vi "Plot XY SM.vi"(0 "Init Plot Cluster":T1={"Y Scale Label Left"="left", "Y Scale Label Right"="right", "X Scale Label"="Time", "Ymin Left"=0.0, "Ymax Left"=1.0, "Ymin Right"=-5.0, "Ymax Right"=5.0, "Number of Left Data"=0, "PlotNames Array"=["Temp1", "Temp2", "Temp3", "Temp4", "Temp5", "Temp6", "Temp7"]}, 2 "Mode":T2, 5 "Add Time":dbl, 7 "Add Data":dbl[](array[numeric])) -> (4 "Plot":cluster{dbl[], dbl[]}[](graph))   [LabVIEW 2014]
uses:
  Dryer Performance/Graph Mode Control.ctl
panel:
  in  "Array":bool[](array[boolean])
  in  "OK":bool
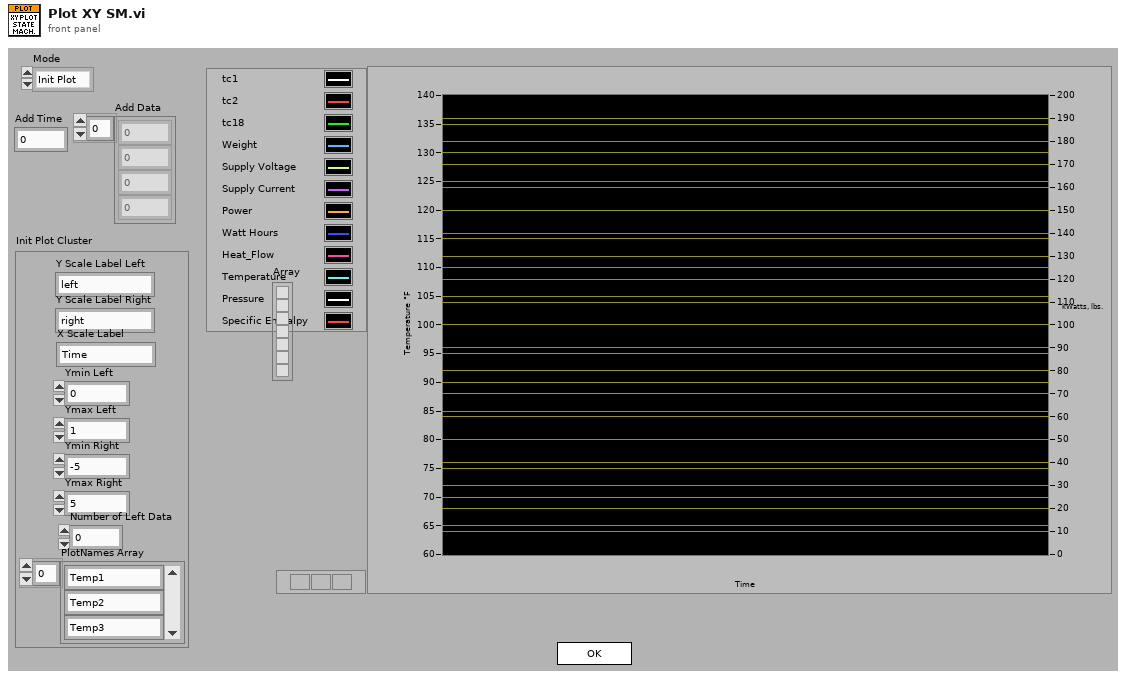
[diagram p1: front panel]
types:
  T1 = cluster{"Y Scale Label Left":string, "Y Scale Label Right":string, "X Scale Label":string, "Ymin Left":dbl, "Ymax Left":dbl, "Ymin Right":dbl, "Ymax Right":dbl, "Number of Left Data":u8, "PlotNames Array":string[]}
  T2 = typedef "Graph Mode Control.ctl" = enum16{"Init Plot", "Add Data", "Simulate"}
  T3 = enum32{"invalid app kind", "Development System", "Run Time System", "Student Edition", "Embedded LabVIEW", "Evaluation", "Custom"}
  T4 = enum32{"Invalid", "Standard", "Closed", "Hidden", "Minimized", "Maximized"}
  T5 = cluster{"Core":cluster{"Current VI Reference":refnum<vi>, "Close Panel on Exit?":bool}, "Num Plots":u32, "Time Array":dbl[], "Data Array":dbl[][], "New Time":dbl, "New Data":dbl[]}
  T6 = cluster{"Current VI Reference":refnum<vi>, "Close Panel on Exit?":bool}
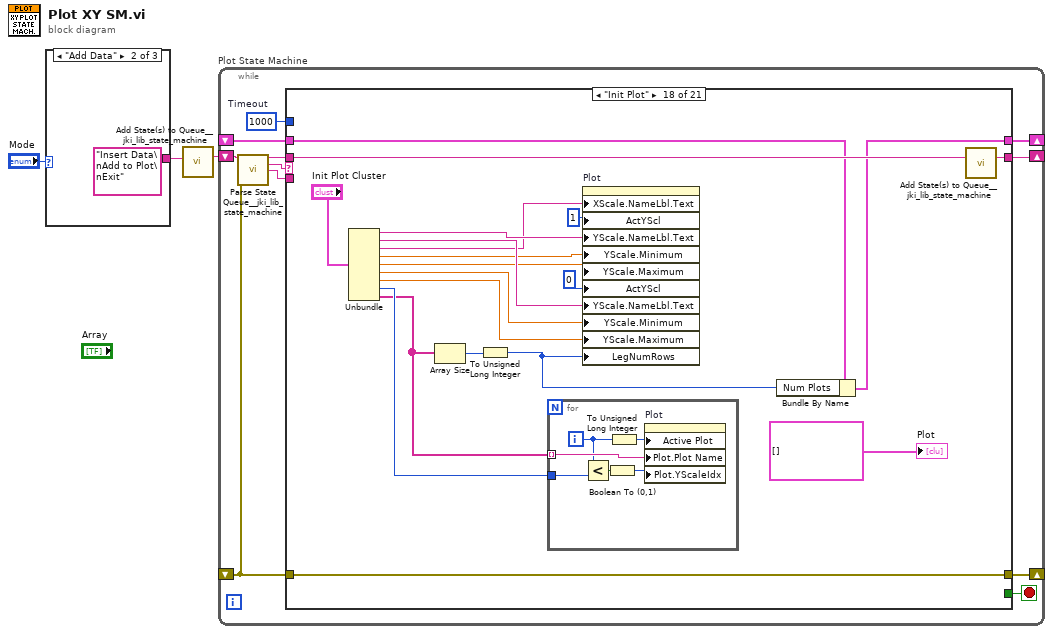
[diagram p0: block diagram]
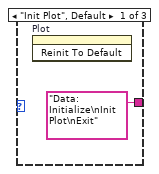
[diagram p2: hidden frame]
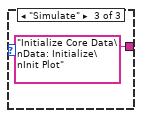
[diagram p3: hidden frame]
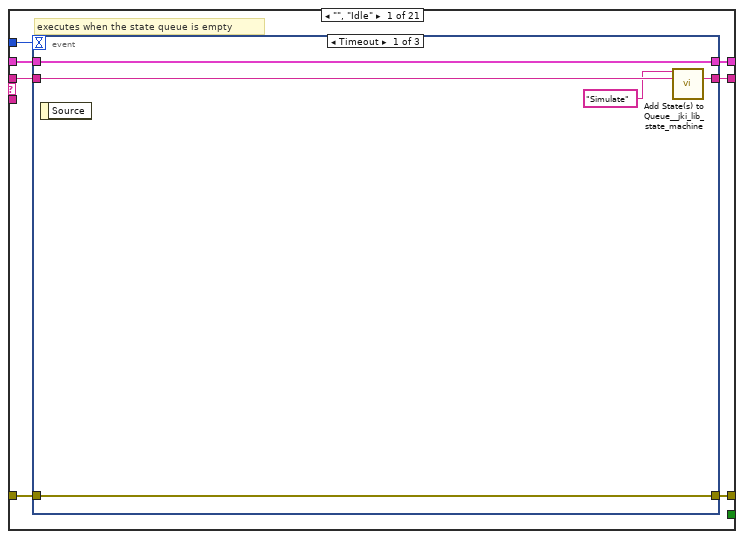
[diagram p4: hidden frame]
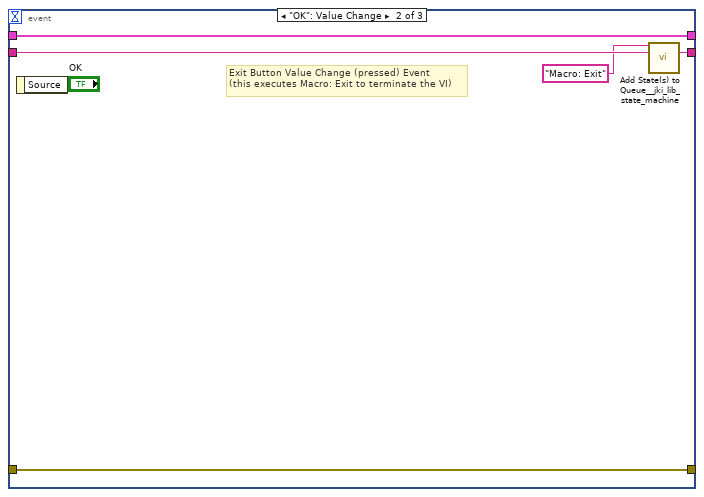
[diagram p5: hidden frame]
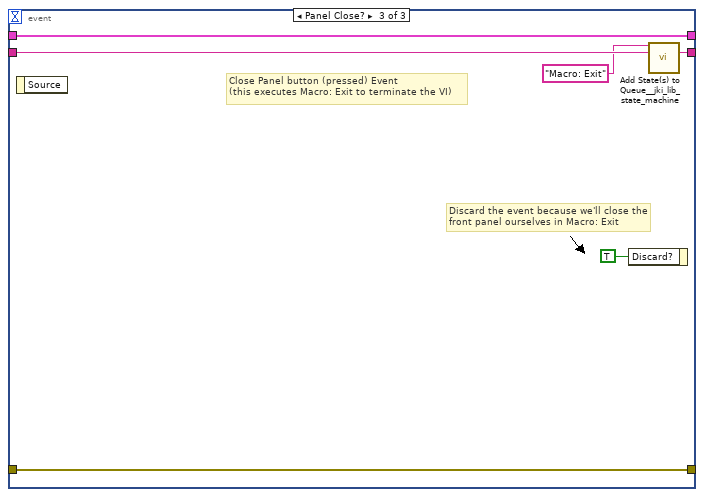
[diagram p6: hidden frame]
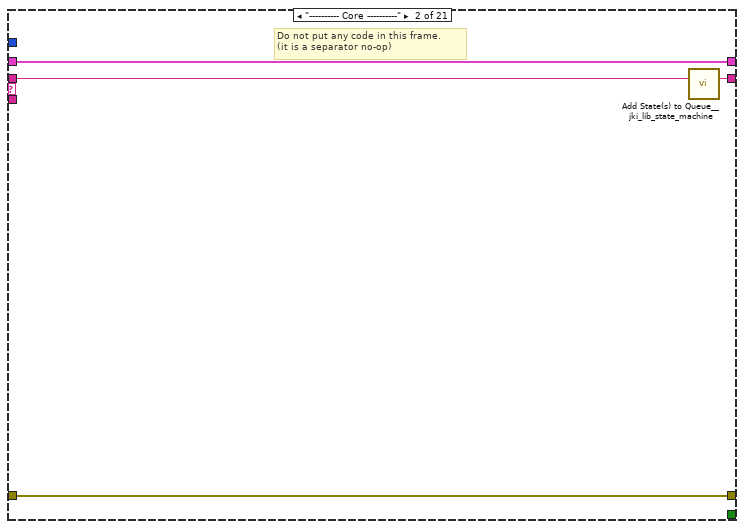
[diagram p7: hidden frame]
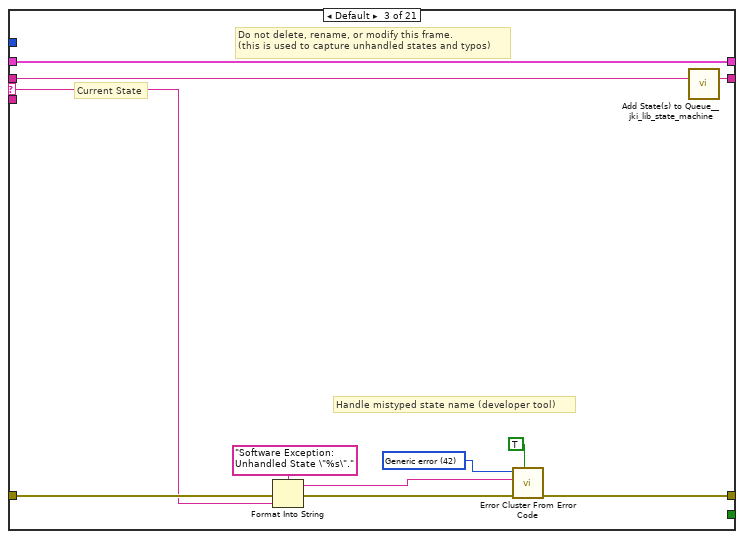
[diagram p8: hidden frame]
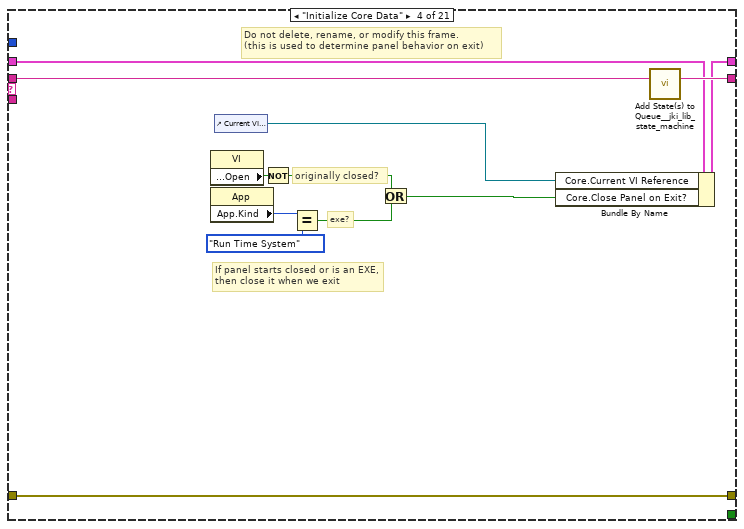
[diagram p9: hidden frame]
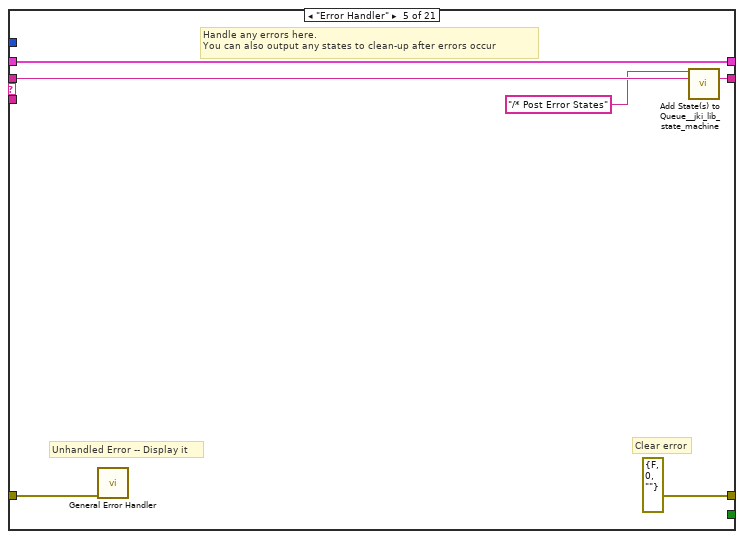
[diagram p10: hidden frame]
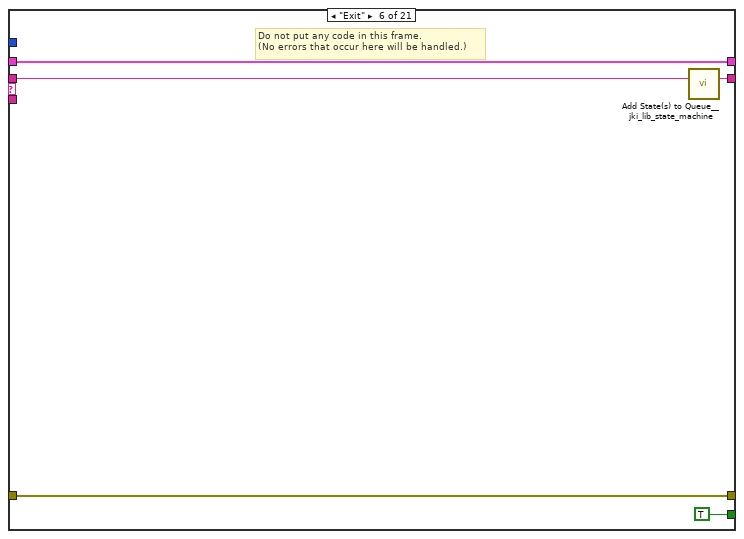
[diagram p11: hidden frame]
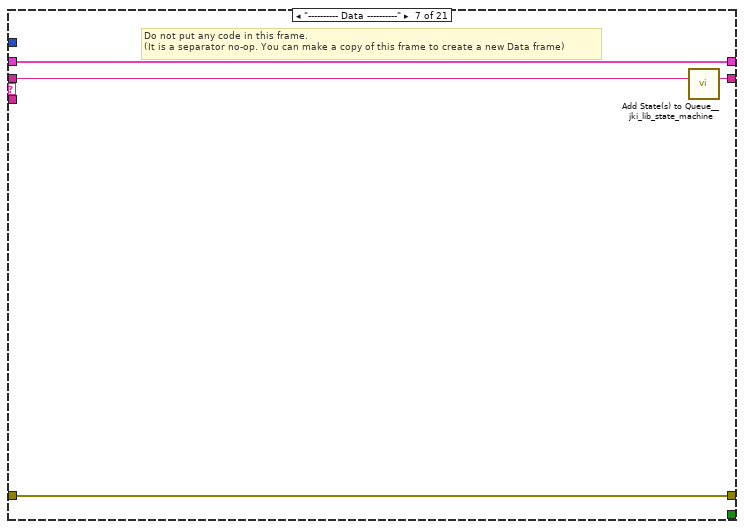
[diagram p12: hidden frame]
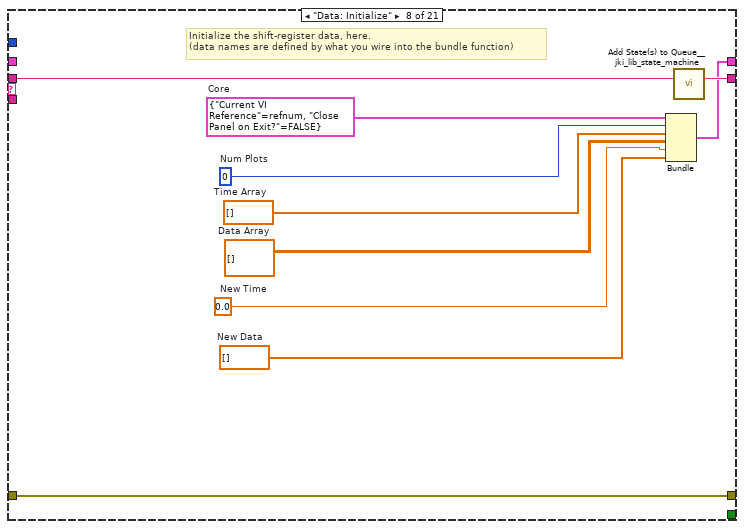
[diagram p13: hidden frame]
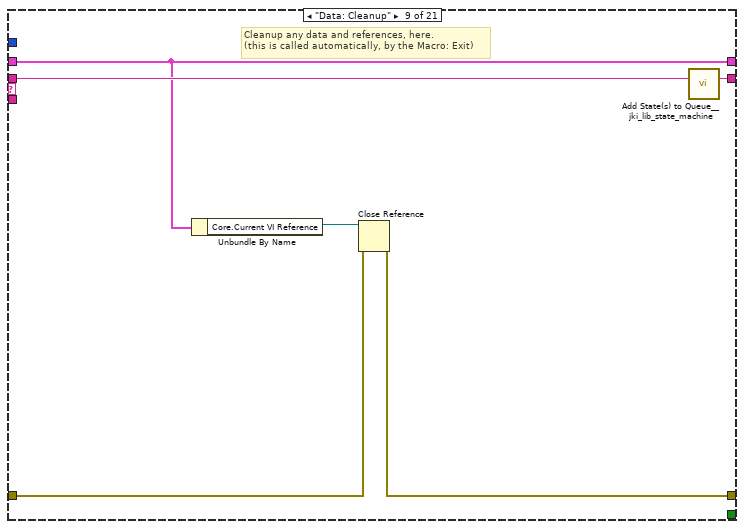
[diagram p14: hidden frame]
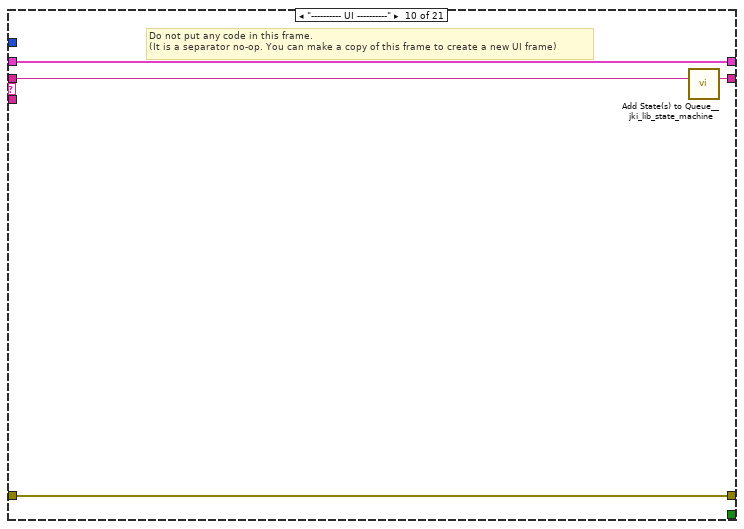
[diagram p15: hidden frame]
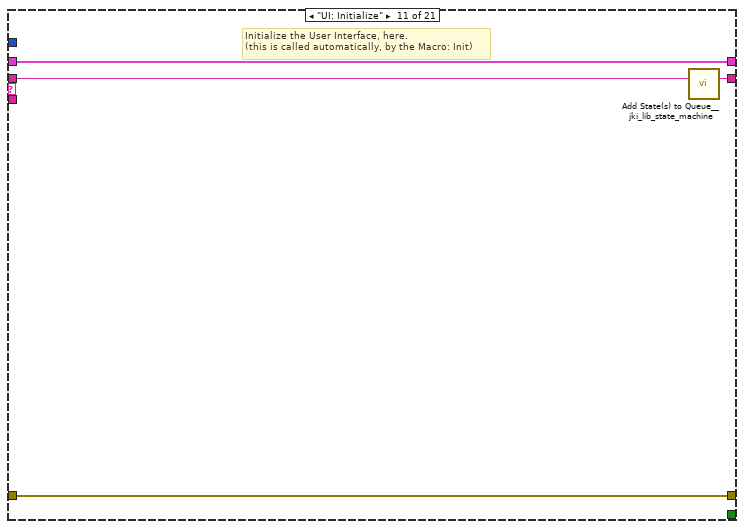
[diagram p16: hidden frame]
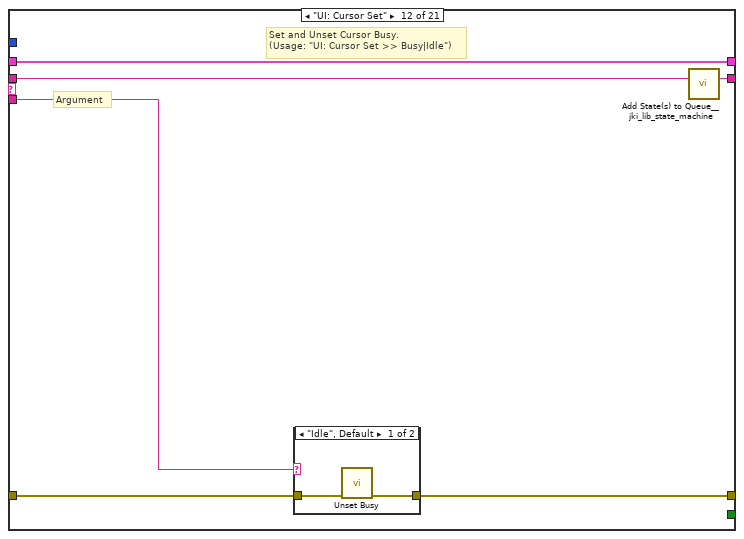
[diagram p17: hidden frame]
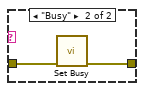
[diagram p18: hidden frame]
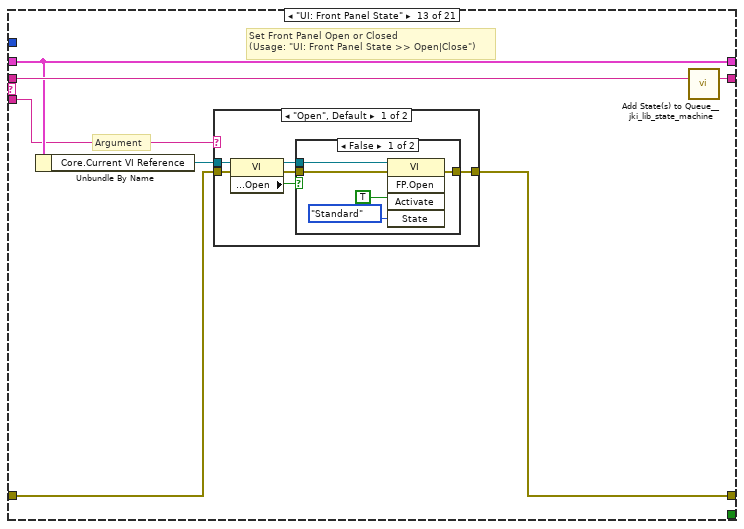
[diagram p19: hidden frame]
diagram:
  n1 = case shown="\"Add Data\"" "Mode" {
    tunnel: ["Data: Initialize\nInit Plot\nExit" "Insert Data\nAdd to Plot\nExit" "Initialize Core Data\nData: Initialize\nInit Plot"] -> w2
    frame "Init Plot", Default {
      n2 = invoke on="Plot" class="XYGraph (strict)" method="Reinit To Default"() -> ()  [unwired: 3 in, 3 out]
    }
    frame "Add Data" {
    }
    frame "Simulate" {
    }
  }
  n3 = call <vilib>:"Add State(s) to Queue__jki_lib_state_machine.vi"("State(s) in (\"\")"=w2) -> ("States Out"=w3:string)  [unwired: 14 in]
  n4 = while "Plot State Machine" {
    shift-right: [w10] -> _
    shift-left: _ -> [w9]
    shift-right: [w13] -> _
    shift-left: _ -> [w7]
    shift-right: [w12] -> _
    shift-left: w3 -> [w14]
    stop <- w11 stop-if-true
    w8 = 1000  # Timeout
    n5 = call <vilib>:"Parse State Queue__jki_lib_state_machine.vi"("State Queue"=w14, "Error In (no error)"=w7) -> ("Remaining States"=w16:string, "Current State"=w17:string, "Arguments"=w15:string)  [unwired: 11 in]
    n6 = case shown="\"Init Plot\"" w17 {
      selector: w17 -> [_ _ w45 _ _ _ _ _ _ _ _ _ _ _ _ _ _ _ _ _ _]
      tunnel: w16 -> [w24 w44 w49 w67 w73 w78 w82 w92 w98 w102 w106 w112 w123 w149 w154 w164 w168 w188 w203 w212 w226]
      tunnel: w15 -> [_ _ _ _ _ _ _ _ _ _ _ w107 w117 _ _ _ _ _ _ _ _]
      tunnel: w9 -> [w22 w41 w47 w58 w70 w76 w79 _ w93 w99 w104 w110 w119 w146 w151 w161 w165 w182 w198 w208 w222]
      tunnel: [w21 w42 w51 w64 errorcluster {"status"=FALSE, "code"=0, "source"=""} ("error out") w75 w80 w89 w94 w100 w103 w108 w120 w147 w152 w162 w166 w186 w201 w210 w224] -> w13
      tunnel: w7 -> [w20 w42 w50 w64 w69 w75 w80 w89 w95 w100 w103 w109 w121 w147 w152 w162 w166 w186 w201 w210 w224]
      tunnel: [w23 w43 w48 w66 w72 w77 w81 w91 w97 w101 w105 w111 w122 w148 w153 w163 w167 w187 w202 w211 w225] -> w12
      tunnel: [_ _ _ _ _ TRUE _ _ _ _ _ _ _ _ _ _ _ _ _ _ _] -> w11
      tunnel: [w19 w41 w47 w65 w70 w76 w79 w90 w93 w99 w104 w110 w119 w146 w151 w161 w165 w181 w197 w207 w221] -> w10
      tunnel: w8 -> [w18 _ _ _ _ _ _ _ _ _ _ _ _ _ _ _ _ _ _ _ _]
      frame "", "Idle" {
        # "executes when the state queue is empty"
        n7 = event shown="[0] Timeout" {
          selector: _ -> [_ _ _]
          dyn-events: _ -> [_ _ _]
          timeout: w18 -> [_ _ _]
          tunnel: w24 -> [w29 w34 w40]
          tunnel: [w28 w33 w39] -> w23
          tunnel: w22 -> [w26 w31 w37]
          tunnel: [w27 w32 w38] -> w21
          tunnel: w20 -> [w27 w32 w38]
          tunnel: [w26 w31 w37] -> w19
          event Timeout {
            n8 = event-data() -> ()  [unwired: 1 in, 1 out]
            n9 = call <vilib>:"Add State(s) to Queue__jki_lib_state_machine.vi"("State(s) in Front (\"\")"="Simulate" ("State(s) in Front (\"\")"), "State(s) in (\"\")"=w29) -> ("States Out"=w28:string)  [unwired: 13 in]
          }
          event "OK": Value Change {
            # "Exit Button Value Change (pressed) Event\n(this executes Macro: Exit to terminate the VI)"
            n10 = event-data() -> ()  [unwired: 1 in, 1 out]
            n11 = call <vilib>:"Add State(s) to Queue__jki_lib_state_machine.vi"("State(s) in Front (\"\")"="Macro: Exit", "State(s) in (\"\")"=w34) -> ("States Out"=w33:string)  [unwired: 13 in]
          }
          event Panel Close? {
            # "Discard the event because we'll close the front panel ourselves in Macro: Exit"
            # "Close Panel button (pressed) Event\n(this executes Macro: Exit to terminate the VI)"
            n12 = event-data() -> ()  [unwired: 1 in, 1 out]
            n13 = event-data("Discard?"=TRUE) -> ()  [unwired: 1 in, 1 out]
            n14 = call <vilib>:"Add State(s) to Queue__jki_lib_state_machine.vi"("State(s) in Front (\"\")"="Macro: Exit", "State(s) in (\"\")"=w40) -> ("States Out"=w39:string)  [unwired: 13 in]
          }
        }
      }
      frame "---------- Core ----------" {
        # "Do not put any code in this frame.\n(it is a separator no-op)"
        n15 = call <vilib>:"Add State(s) to Queue__jki_lib_state_machine.vi"("State(s) in (\"\")"=w44) -> ("States Out"=w43:string)  [unwired: 14 in]
      }
      frame Default {
        w54 = 42 items=["No error", "Argument error", "Memory is full", "Out of zone", "End of file", "File already open", "Generic file I/O error", "File not found", "File permission error", "Disk is full", "Duplicate path", "Too many files open", "System feature not enabled", "Resource file not found", "Cannot add resource", "Resource not found", "Image not found", "Image memory error", "Pen does not exist", "Config type invalid", "Config token not found", "Config parse error", "Config memory error", "Bad external code format", "Bad external code offset", "External code not present", "Null window", "Destroy window error", "Null menu", "Print aborted", "Bad print record", "Print driver error", "Windows error during printing", "Memory error during printing", "Print dialog error", "Generic print error", "Invalid device refnum", "Device not found", "Device parameter error", "Device unit error", "Cannot open device", "Device call aborted", "Generic error", "Cancelled by user", "Object ID too low", "Object ID too high", "Object not in heap", "Unknown heap", "Unknown object (invalid DefProc)", "Unknown object (DefProc not in table)", "Message out of range", "Invalid (null) method", "Unknown message", "Manager call not supported", "Bad address", "Network operation in progress", "Network operation timed out", "Connection is busy", "Network attribute not supported", "Network error", "Address in use", "System out of memory", "Connection aborted", "Connection refused", "Not connected", "Already connected", "Connection closed", "Initialization error (interapplication manager)", "Bad occurrence", "Wait on unbound occurrence handler", "Occurrence queue overflow", "Datalog type conflict", "Unused", "Unrecognized type (interapplication manager)", "Memory corrupt", "Failed to make temporary DLL", "Old CIN version", "Drag socket not found", "Failed to load drop-object", "Failed to register OLE object", "Failed to release OLE object", "Format specifier type mismatch", "Unknown format specifier", "Too few format specifiers", "Too many format specifiers", "Scan failed", "Newer CIN version", "Error converting to variant", "Runtime menu error", "Password tampered", "Variant attribute not found", "Incompatible variant data type", "Event data is not available", "Event Store is not present", "Occurrence is not found", "Event Queue is not created", "Event info is not available", "Refnum passed is NULL", "Error retrieving Class GUID", "Error retrieving CoClass GUID", "Error retrieving TypeLib GUID.", "Bad built application magic bytes.", "Specific driver is different from the specific driver associated with the Logical Name.", "There is no session opened to the class driver.", "Max Error", "MAX - Error with config objects", "MAX - Error loading configuration", "MAX - Group not supported"]
        # "Current State"
        # "Do not delete, rename, or modify this frame.\n(this is used to capture unhandled states and typos)"
        # "Handle mistyped state name (developer tool)"
        n16 = Format Into String(format string="Software Exception: Unhandled State \"%s\"." ("message"), error in=w50, w45) -> (resulting string=w53:string, error out=w52:errorcluster)  [unwired: 1 in]
        n17 = call <vilib>:"Error Cluster From Error Code.vi"("show call chain? (False)"=TRUE, "error in (no error)"=w52, "error message (\"\")"=w53, "error code (0)"=w54) -> ("error out"=w51:errorcluster)  [unwired: 5 in]
        n18 = call <vilib>:"Add State(s) to Queue__jki_lib_state_machine.vi"("State(s) in (\"\")"=w49) -> ("States Out"=w48:string)  [unwired: 14 in]
      }
      frame "Initialize Core Data" {
        # "Do not delete, rename, or modify this frame.\n(this is used to determine panel behavior on exit)"
        # "originally closed?"
        # "exe?"
        # "If panel starts closed or is an EXE, then close it when we exit"
        n19 = property class="VI"() -> ("Front Panel.Open"=w63:bool)  [unwired: 2 in, 2 out]
        n20 = property class="App"() -> ("App.Kind"=w62:T3)  [unwired: 2 in, 2 out]
        n21 = control-ref of="Current VI Reference"() -> (w56:refnum<vi>)
        n22 = Not(x=w63) -> (.not. x?=w60:bool)
        n23 = Equal?(x=w62, y=T3."Run Time System" ("Application:Kind")) -> (x = y?=w59:bool)
        n24 = Or(x=w60, y=w59) -> (x .or. y?=w57:bool)
        n25 = Bundle By Name(cluster=w58, "Core.Current VI Reference"=w56, "Core.Close Panel on Exit?"=w57) -> (w65:T5)
        n26 = call <vilib>:"Add State(s) to Queue__jki_lib_state_machine.vi"("State(s) in (\"\")"=w67) -> ("States Out"=w66:string)  [unwired: 14 in]
      }
      frame "Error Handler" {
        # "Unhandled Error -- Display it"
        # "Handle any errors here.\nYou can also output any states to clean-up after errors occur"
        # "Clear error"
        n27 = call <vilib>:"General Error Handler.vi"("error in (no error)"=w69) -> ()  [unwired: 10 in, 5 out]
        n28 = call <vilib>:"Add State(s) to Queue__jki_lib_state_machine.vi"("State(s) in Front (\"\")"="/* Post Error States", "State(s) in (\"\")"=w73) -> ("States Out"=w72:string)  [unwired: 13 in]
      }
      frame "Exit" {
        # "Do not put any code in this frame.\n(No errors that occur here will be handled.)"
        n29 = call <vilib>:"Add State(s) to Queue__jki_lib_state_machine.vi"("State(s) in (\"\")"=w78) -> ("States Out"=w77:string)  [unwired: 14 in]
      }
      frame "---------- Data ----------" {
        # "Do not put any code in this frame.\n(It is a separator no-op. You can make a copy of this frame to create a new Data frame)"
        n30 = call <vilib>:"Add State(s) to Queue__jki_lib_state_machine.vi"("State(s) in (\"\")"=w82) -> ("States Out"=w81:string)  [unwired: 14 in]
      }
      frame "Data: Initialize" {
        w84 = 0.0  # New Time
        w83 = dbl[] []  # New Data
        w85 = dbl[][] []  # Data Array
        w86 = dbl[] []  # Time Array
        w87 = T6 {"Current VI Reference"=refnum, "Close Panel on Exit?"=FALSE}  # Core
        w88 = u32 0  # Num Plots
        # "Initialize the shift-register data, here.\n(data names are defined by what you wire into the bundle function)"
        n31 = Bundle("Core"=w87, "Num Plots"=w88, "Time Array"=w86, "Data Array"=w85, "New Time"=w84, "New Data"=w83) -> (w90:T5)  [unwired: 1 in]
        n32 = call <vilib>:"Add State(s) to Queue__jki_lib_state_machine.vi"("State(s) in (\"\")"=w92) -> ("States Out"=w91:string)  [unwired: 14 in]
      }
      frame "Data: Cleanup" {
        # "Cleanup any data and references, here.\n(this is called automatically, by the Macro: Exit)"
        n33 = Unbundle By Name(w93) -> ("Core.Current VI Reference"=w96:refnum<vi>)
        n34 = Close Reference(reference=w96, error in (no error)=w95) -> (error out=w94:errorcluster)
        n35 = call <vilib>:"Add State(s) to Queue__jki_lib_state_machine.vi"("State(s) in (\"\")"=w98) -> ("States Out"=w97:string)  [unwired: 14 in]
      }
      frame "---------- UI ----------" {
        # "Do not put any code in this frame.\n(It is a separator no-op. You can make a copy of this frame to create a new UI frame)"
        n36 = call <vilib>:"Add State(s) to Queue__jki_lib_state_machine.vi"("State(s) in (\"\")"=w102) -> ("States Out"=w101:string)  [unwired: 14 in]
      }
      frame "UI: Initialize" {
        # "Initialize the User Interface, here.\n(this is called automatically, by the Macro: Init)"
        n37 = call <vilib>:"Add State(s) to Queue__jki_lib_state_machine.vi"("State(s) in (\"\")"=w106) -> ("States Out"=w105:string)  [unwired: 14 in]
      }
      frame "UI: Cursor Set" {
        # "Argument"
        # "Set and Unset Cursor Busy.\n(Usage: \"UI: Cursor Set >> Busy|Idle\")"
        n38 = case shown="\"Idle\", Default" w107 {
          tunnel: w109 -> [w114 w116]
          tunnel: [w113 w115] -> w108
          frame "Idle", Default {
            n39 = call <vilib>:"Unset Busy.vi"("error in (no error)"=w114) -> ("error out"=w113:errorcluster)  [unwired: 10 in]
          }
          frame "Busy" {
            n40 = call <vilib>:"Set Busy.vi"("error in (no error)"=w116) -> ("error out"=w115:errorcluster)  [unwired: 9 in, 1 out]
          }
        }
        n41 = call <vilib>:"Add State(s) to Queue__jki_lib_state_machine.vi"("State(s) in (\"\")"=w112) -> ("States Out"=w111:string)  [unwired: 14 in]
      }
      frame "UI: Front Panel State" {
        # "Argument"
        # "Set Front Panel Open or Closed\n(Usage: \"UI: Front Panel State >> Open|Close\")"
        n42 = Unbundle By Name(w119) -> ("Core.Current VI Reference"=w118:refnum<vi>)
        n43 = case shown="\"Open\", Default" w117 {
          tunnel: w121 -> [w127 w140]
          tunnel: [w129 w141] -> w120
          tunnel: w118 -> [w128 w138]
          frame "Open", Default {
            n44 = property class="VI"(reference=w128, error in=w127) -> (reference out=w125:refnum<vi>, error out=w126:errorcluster, "Front Panel.Open"=w124:bool)
            n45 = case shown="False" w124 {
              tunnel: [w132 w135] -> w129
              tunnel: w126 -> [w131 w135]
              tunnel: w125 -> [w130 _]
              frame False {
                n46 = invoke class="VI" method="FP.Open"(reference=w130, error in=w131, "Activate"=TRUE, "State"=T4."Standard") -> (error out=w132:errorcluster)  [unwired: 1 in, 4 out]
              }
              frame True {
              }
            }
          }
          frame "Close" {
            n47 = property class="VI"(reference=w138, error in=w140) -> (reference out=w137:refnum<vi>, error out=w139:errorcluster, "Front Panel.Open"=w136:bool)
            n48 = case shown="True" w136 {
              tunnel: [w142 w145] -> w141
              tunnel: w139 -> [w142 w144]
              tunnel: w137 -> [_ w143]
              frame False {
              }
              frame True {
                n49 = invoke class="VI" method="FP.Close"(reference=w143, error in=w144) -> (error out=w145:errorcluster)  [unwired: 1 in, 2 out]
              }
            }
          }
        }
        n50 = call <vilib>:"Add State(s) to Queue__jki_lib_state_machine.vi"("State(s) in (\"\")"=w123) -> ("States Out"=w122:string)  [unwired: 14 in]
      }
      frame "---------- Macro ----------" {
        # "Do not put any code in this frame.\n(It is a separator no-op. You can make a copy of this frame to create a new Macro frame)"
        n51 = call <vilib>:"Add State(s) to Queue__jki_lib_state_machine.vi"("State(s) in (\"\")"=w149) -> ("States Out"=w148:string)  [unwired: 14 in]
      }
      frame "Macro: Initialize" {
        w150 = "Data: Initialize\nInitialize Core Data\nUI: Initialize\nUI: Front Panel State >> Open"  # Data: Initialize Initialize Core Data UI: Initialize UI: Front Panel State >> Open
        # "Initialization Macro\n(This is called once, when the VI starts)"
        n52 = call <vilib>:"Add State(s) to Queue__jki_lib_state_machine.vi"("State(s) in Front (\"\")"=w150, "State(s) in (\"\")"=w154) -> ("States Out"=w153:string)  [unwired: 13 in]
      }
      frame "Macro: Exit" {
        # "Exit Macro\n(This is called once, when the VI exits)"
        n53 = Unbundle By Name(w161) -> ("Core.Close Panel on Exit?"=w160:bool)
        n54 = Select(t="UI: Front Panel State >> Close", s=w160, f="") -> (s? t:f=w157:string)
        n55 = call <vilib>:"Add State(s) to Queue__jki_lib_state_machine.vi"("State(s) in (\"\")"=w157, "State(s) at Back (\"\")"="Data: Cleanup\nExit") -> ("States Out"=w155:string)  [unwired: 13 in]
        n56 = call <vilib>:"Add State(s) to Queue__jki_lib_state_machine.vi"("State(s) in Front (\"\")"=w155, "State(s) in (\"\")"=w164) -> ("States Out"=w163:string)  [unwired: 13 in]
      }
      frame "---------- New Category ----------" {
        # "Template Separator\n(You can make a copy of, or modify, this frame)"
        n57 = call <vilib>:"Add State(s) to Queue__jki_lib_state_machine.vi"("State(s) in (\"\")"=w168) -> ("States Out"=w167:string)  [unwired: 14 in]
      }
      frame "Init Plot" {
        n58 = Unbundle("Init Plot Cluster") -> ("Y Scale Label Left"=w177:string, "Y Scale Label Right"=w176:string, "X Scale Label"=w175:string, "Ymin Left"=w174:dbl, "Ymax Left"=w173:dbl, "Ymin Right"=w172:dbl, "Ymax Right"=w171:dbl, "Number of Left Data"=w170:u8, "PlotNames Array"=w169:string[])
        n59 = Array Size(array=w169) -> (size(s)=w184:i32)
        n60 = To Unsigned Long Integer(number=w184) -> (unsigned 32bit integer=w179:u32)
        n61 = for {
          tunnel: w169 -> [w194] mode=indexing
          tunnel: w170 -> [w191]
          i -> [w192]
          n62 = Less?(x=w192, y=w191) -> (x < y?=w189:bool)
          n63 = Boolean To (0,1)(Boolean=w189) -> (0, 1=w190:i16)
          n64 = To Unsigned Long Integer(number=w192) -> (unsigned 32bit integer=w193:u32)
          n65 = property on="Plot" class="XYGraph (strict)"("Active Plot"=w193, "Plot.Plot Name"=w194, "Plot.YScaleIdx"=w190) -> ()  [unwired: 2 in, 2 out]
        }
        n66 = property on="Plot" class="XYGraph (strict)"("XScale.NameLbl.Text"=w175, "ActYScl"=1 ("Active Y Scale"), "YScale.NameLbl.Text"=w177, "YScale.Minimum"=w174, "YScale.Maximum"=w173, "ActYScl"=0 ("Active Y Scale"), "YScale.NameLbl.Text"=w176, "YScale.Minimum"=w172, "YScale.Maximum"=w171, "LegNumRows"=w179) -> ()  [unwired: 2 in, 2 out]
        n67 = Bundle By Name(cluster=w182, "Num Plots"=w179) -> (w181:T5)
        n68 = call <vilib>:"Add State(s) to Queue__jki_lib_state_machine.vi"("State(s) in (\"\")"=w188) -> ("States Out"=w187:string)  [unwired: 14 in]
        "Plot" <- cluster{dbl[], dbl[]}[] [] ("RHS Tank TCs")
      }
      frame "Simulate" {
        n69 = Unbundle By Name(w198) -> ("Num Plots"=w200:u32)
        n70 = for {
          N: w200 -> [_]
          tunnel: [w204] -> w195 mode=indexing
          n71 = Random Number (0-1)() -> (number: 0 to 1=w204:dbl)
        }
        n72 = call "UTILITY E-Time.vi"() -> ("Elapsed Time (sec)"=w196:dbl)  [unwired: 9 in, 2 out]
        n73 = Bundle By Name(cluster=w198, "New Time"=w196, "New Data"=w195) -> (w197:T5)
        n74 = call <vilib>:"Add State(s) to Queue__jki_lib_state_machine.vi"("State(s) in Front (\"\")"="Add to Plot" ("State(s) in Front (\"\")"), "State(s) in (\"\")"=w203) -> ("States Out"=w202:string)  [unwired: 13 in]
      }
      frame "Insert Data" {
        n75 = Bundle By Name(cluster=w208, "New Time"="Add Time", "New Data"="Add Data") -> (w207:T5)
        n76 = call <vilib>:"Add State(s) to Queue__jki_lib_state_machine.vi"("State(s) in Front (\"\")"="Add to Plot" ("State(s) in Front (\"\")"), "State(s) in (\"\")"=w212) -> ("States Out"=w211:string)  [unwired: 13 in]
      }
      frame "Add to Plot" {
        # "Your code here.\n(You can make a copy of, or modify, this frame)"
        n77 = Unbundle By Name(w222) -> ("New Time"=w216:dbl, "New Data"=w213:dbl[], "Time Array"=w215:dbl[], "Data Array"=w219:dbl[][])
        n78 = Transpose 2D Array(2D array=w219) -> (transposed array=w214:dbl[][])
        n79 = Build Array (concatenate)(w215, w216) -> (w220:dbl[])
        n80 = Build Array (concatenate)(w214, w213) -> (w218:dbl[][])
        n81 = Transpose 2D Array(2D array=w218) -> (transposed array=w217:dbl[][])
        n82 = for {
          tunnel: w220 -> [w229]
          tunnel: [w228] -> w223 mode=indexing
          tunnel: w217 -> [w227] mode=indexing
          n83 = Bundle(w229, w227) -> (w228:cluster{dbl[], dbl[]})  [unwired: 1 out]
        }
        n84 = local write "Plot"(w223) -> ()
        n85 = Bundle By Name(cluster=w222, "Time Array"=w220, "Data Array"=w217) -> (w221:T5)
        n86 = call <vilib>:"Add State(s) to Queue__jki_lib_state_machine.vi"("State(s) in (\"\")"=w226) -> ("States Out"=w225:string)  [unwired: 14 in]
      }
    }
  }
